vi "MB Serial Slave Communication.vi"(6 "Data Reference":T1, 8 "error in (no error)":errorcluster, 9 "Timeout":u32=10000, 10 "Serial Parameters":T2 {"Slave Address" format="%.0x"}, 11 "VISA resource name":refnum<visa-resource-name>) -> (0 "error out":errorcluster, 3 "VISA resource name out":refnum<visa-resource-name>)   [LabVIEW 2019, in "NI_modbus_upd.lvlib"]
uses:
  NI_modbus_upd.lvlib
panel:
  # "VI Name: MB Serial Slave Communication.vi\nPurpose: MODBUS Slave Read."
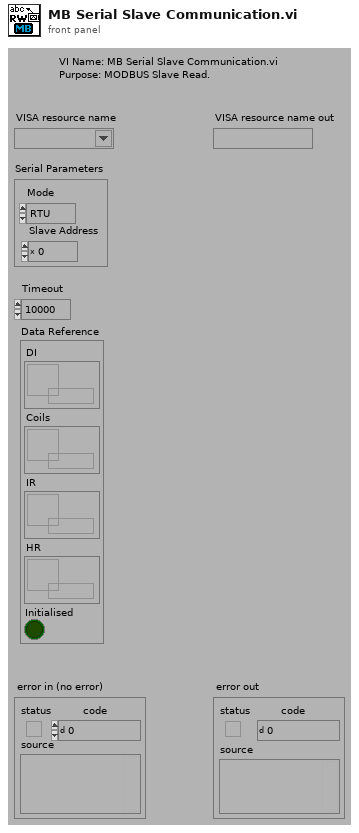
[diagram p1: front panel]
types:
  T1 = cluster{"DI":refnum<data-value>, "Coils":refnum<data-value>, "IR":refnum<data-value>, "HR":refnum<data-value>, "Initialised":bool}
  T2 = cluster{"Mode":enum16{"RTU", "ASCII"}, "Slave Address":u8}
  T3 = typedef "NI_modbus_upd.lvlib/MB Modbus Data Unit.ctl" = cluster{"function":T4, "Data":u8[]}
  T4 = typedef "NI_modbus_upd.lvlib/Function.ctl" = u8
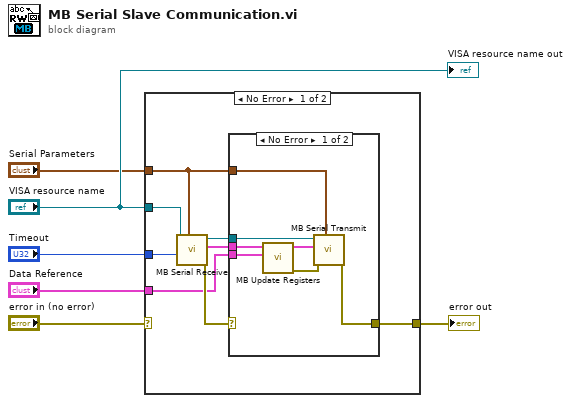
[diagram p0: block diagram]
diagram:
  n1 = case shown="No Error" "error in (no error)" {
    selector: "error in (no error)" -> [_ w23]
    tunnel: "VISA resource name" -> [w14 _]
    tunnel: [w13 w23] -> w6
    tunnel: "Timeout" -> [w11 _]
    tunnel: "Serial Parameters" -> [w8 _]
    tunnel: "Data Reference" -> [w7 _]
    frame No Error {
      n2 = call "MB Serial Receive.vi"("Serial Parameters"=w8, "Timeout"=w11, "VISA resource name"=w14) -> ("error out"=w9:errorcluster, "Modbus Data Unit"=w10:T3, "VISA resource name out"=w12:refnum<visa-resource-name>)  [unwired: 5 in, 1 out]
      n3 = case shown="No Error" w9 {
        selector: w9 -> [_ w22]
        tunnel: [w21 w22] -> w13
        tunnel: w12 -> [w20 _]
        tunnel: w8 -> [w18 _]
        tunnel: w10 -> [w17 _]
        tunnel: w7 -> [w15 _]
        frame No Error {
          n4 = call "MB Update Registers.vi"("Data Reference"=w15, "Modbus Data Unit In"=w17) -> ("error out"=w19:errorcluster, "Modbus Data Unit Out"=w16:T3)  [unwired: 8 in]
          n5 = call "MB Serial Transmit.vi"("Serial Parameters"=w18, "error in (no error)"=w19, "Modbus Data Unit"=w16, "VISA resource name"=w20) -> ("error out"=w21:errorcluster)  [unwired: 6 in, 1 out]
        }
        frame Error {
        }
      }
    }
    frame Error {
    }
  }
  "error out" <- w6
  "VISA resource name out" <- "VISA resource name"
